vi "D2SParser - Private - Function - Read Skills.vi"(8 "error in (no error)":errorcluster, 11 "D2SParser in":refnum<class "D2SParser.lvclass">) -> (0 "error out":errorcluster, 3 "D2SParser out":refnum<class "D2SParser.lvclass">)   [LabVIEW 2015, in "D2SParser.lvclass"]
uses:
  D2SParser.lvclass
  D2SParser.lvclass/D2SParser.ctl
  D2Character/D2Character.lvclass/D2Character.ctl
  D2Character/D2Character - Accessors - Get Skills.vi
  D2Character/D2Character - Accessors - Set Skills.vi
  D2SkillsTable/D2SkillsTable.lvclass
  D2Character/D2Character.lvclass
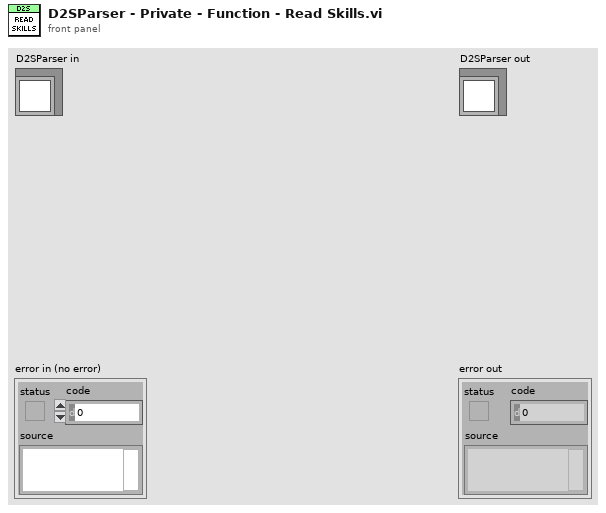
[diagram p1: front panel]
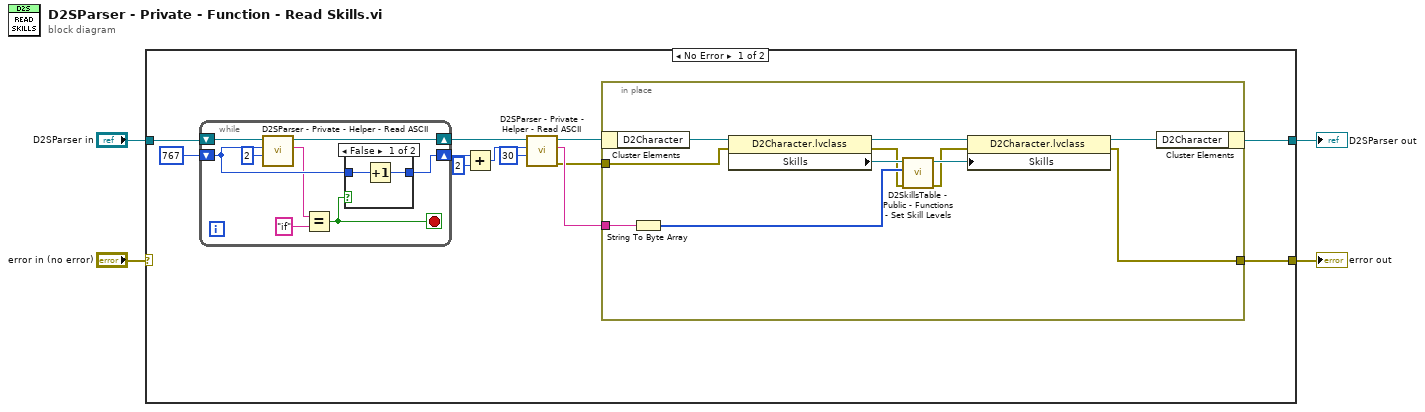
[diagram p0: block diagram]
diagram:
  n1 = case shown="No Error" "error in (no error)" {
    selector: "error in (no error)" -> [_ w40]
    tunnel: [w16 w40] -> w3
    tunnel: [w15 w39] -> w1
    tunnel: "D2SParser in" -> [w13 w39]
    frame No Error {
      n2 = while {
        shift-right: [w22] -> w10
        shift-left: i64 767 ("Position") -> [w23]
        shift-right: [w17] -> w12
        shift-left: w13 -> [w24]
        stop <- w18 stop-if-true
        n3 = call "D2SParser - Private - Helper - Read ASCII.vi"("# Characters"=2, "Position"=w23, "D2SParser in"=w24) -> ("ASCII"=w20:string, "D2SParser out"=w17:refnum<class "D2SParser.lvclass">)  [unwired: 6 in, 1 out]
        n4 = Equal?(x=w20, y="if") -> (x = y?=w18:bool)
        n5 = case shown="False" w18 {
          tunnel: w23 -> [w26 w27]
          tunnel: [w25 w27] -> w22
          frame False {
            n6 = Increment(x=w26) -> (x+1=w25:i64)
          }
          frame True {
          }
        }
      }
      n7 = Add(x=w10, y=i64 2) -> (x+y=w9:i64)
      n8 = call "D2SParser - Private - Helper - Read ASCII.vi"("# Characters"=30, "Position"=w9, "D2SParser in"=w12) -> ("error out"=w5:errorcluster, "ASCII"=w6:string, "D2SParser out"=w11:refnum<class "D2SParser.lvclass">)  [unwired: 6 in]
      n9 = in-place {
        in-place-border: [w33] -> w16
        in-place-border: w6 -> [w37]
        in-place-border: w5 -> [w36]
        n10 = in-place-cluster #1(w11) -> ("D2Character"=w38:refnum<class "D2Character.lvclass">)
        n11 = String To Byte Array(string=w37) -> (unsigned byte array=w30:u8[])
        n12 = property class="D2Character.lvclass"(reference=w38, error in=w36) -> (reference out=w35:refnum<class "D2Character.lvclass">, error out=w29:errorcluster, "Skills"=w32:refnum<class "D2SkillsTable.lvclass">)
        n13 = call "D2SkillsTable - Public - Functions - Set Skill Levels.vi"("error in (no error)"=w29, "Levels"=w30, "D2SkillsTable in"=w32) -> ("error out"=w28:errorcluster, "D2SkillsTable out"=w31:refnum<class "D2SkillsTable.lvclass">)  [unwired: 7 in]
        n14 = property class="D2Character.lvclass"(reference=w35, error in=w28, "Skills"=w31) -> (reference out=w34:refnum<class "D2Character.lvclass">, error out=w33:errorcluster)
        n15 = in-place-cluster #1("D2Character"=w34) -> (w15:refnum<class "D2SParser.lvclass">)
      }
    }
    frame Error {
    }
  }
  "error out" <- w3
  "D2SParser out" <- w1
